vi "Мультиплексор5.vi"(1 "C":bool, 2 "X1":T2, 3 "X0":T3) -> (0 "Y":T1)   [LabVIEW 2017]
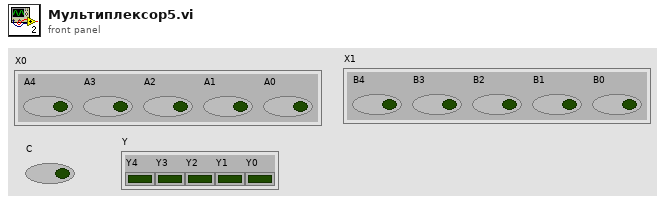
[diagram p1: front panel]
types:
  T1 = cluster{"Y4":bool, "Y3":bool, "Y2":bool, "Y1":bool, "Y0":bool}
  T2 = cluster{"B4":bool, "B3":bool, "B2":bool, "B1":bool, "B0":bool}
  T3 = cluster{"A4":bool, "A3":bool, "A2":bool, "A1":bool, "A0":bool}
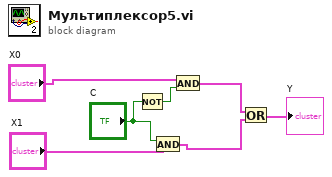
[diagram p0: block diagram]
diagram:
  n1 = Not(x="C") -> (.not. x?=w7:bool)
  n2 = And(x="C", y="X1") -> (x .and. y?=w3:T2)
  n3 = And(x="X0", y=w7) -> (x .and. y?=w4:T3)
  n4 = Or(x=w4, y=w3) -> (x .or. y?=→"Y":cluster{bool, bool, bool, bool, bool})
